vi "Get Anchor Coordinates.vi"(8 "error in (no error)":errorcluster, 10 "Raw Coords":cluster{"X":i32, "Y":i32}, 11 "Shape in":refnum<class "Shape.lvclass">) -> (0 "error out":errorcluster, 2 "Anchor Coords":cluster{dbl, dbl}, 3 "Shape out":refnum<class "Shape.lvclass">)   [LabVIEW 2015, in "LV Image Editor Framework.lvlib" / "Shape.lvclass"]
uses:
  Shape.lvclass
  Shape.lvclass/Shape.ctl
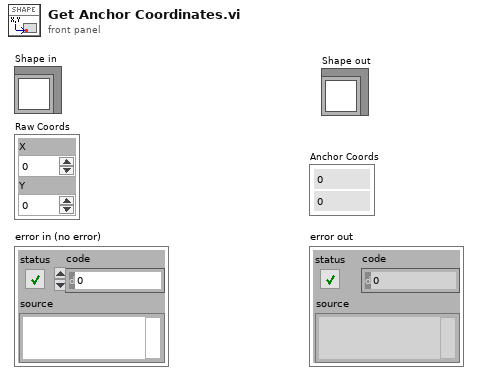
[diagram p1: front panel]
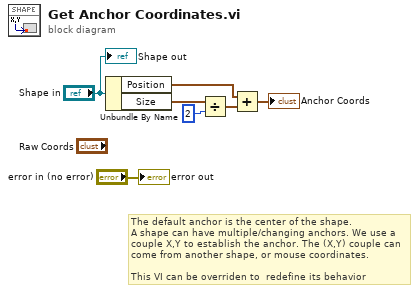
[diagram p0: block diagram]
diagram:
  # "The default anchor is the center of the shape.\nA shape can have multiple/changing anchors. We use a couple X,Y to establish the anchor. The (X,Y) couple can come from another shape, or mouse coordinates. \n\nThis VI can be overriden to  redefine its behavior"
  n1 = Unbundle By Name("Shape in") -> ("Position"=w5:cluster{"Left":i32, "Top":i32}, "Size"=w6:cluster{"Width":i32, "Height":i32})
  n2 = Divide(x=w6, y=2) -> (x/y=w3:cluster{"Width":dbl, "Height":dbl})
  n3 = Add(x=w5, y=w3) -> (x+y=→"Anchor Coords":cluster{dbl, dbl})
  "Shape out" <- "Shape in"
  "error out" <- "error in (no error)"
